vi "SetAttributeViString.vi"(7 "AttributeValue":string, 8 "error in (no error)":errorcluster {"code" format="%.0x"}, 9 "AttributeID":u32(ring)=1150015 items=["CALIBRATION_MESSAGE"=1150015, "CALIBRATION_SECURITY_CODE "=1150013, "DIGITIZER_MEMORY_MEASUREMENT_DATA_AUTO_SAVE_FILE"=1150071, "DISPLAY_TEXT"=1150017, "ROUTE_MONITOR_CHANNEL"=1150010, "SCAN_LIST"=1150004, "SYSTEM_DATE"=1150020, "SYSTEM_TIME"=1150021, "SYSTEM_TRACING_FILE_NAME"=1150042, "USB_MEMORY_DATA_FILE"=1150056, "USB_MEMORY_MEASUREMENTS_DATA_AUTO_SAVE_FILE"=1150058, "USB_MEMORY_SELECT_RECALL_AUTO_FILE"=1150053], 11 "instrument handle":refnum<k15>) -> (0 "error out":errorcluster {"code" format="%.0x"}, 3 "instrument handle out":refnum<k15>)   [LabVIEW 2020, in "Keysight DAQ970.lvlib"]
doc: "Sets a String attribute from the instrument driver.\nThe following Attributes are supported:\n\nCALIBRATION_MESSAGE\n\nCALIBRATION_SECURITY_CODE\n\nDIGITIZER_MEMORY_MEASUREMENT_DATA_AUTO_SAVE_FILE\n\nDISPLAY_TEXT\n\nROUTE_MONITOR_CHANNEL\n\nSCAN_LIST\n\nSYSTEM_DATE\n\nSYSTEM_TIME\n\nSYSTEM_TRACING_FILE_NAME\n\nUSB_MEMORY_DATA_FILE\n\nUSB_MEMORY_MEASUREMENTS_DATA_AUTO_SAVE_FILE\n\nUSB_MEMORY_SELECT_RECALL_AUTO_FILE"
uses:
  Keysight DAQ970.lvlib
  KtDAQ970.dll
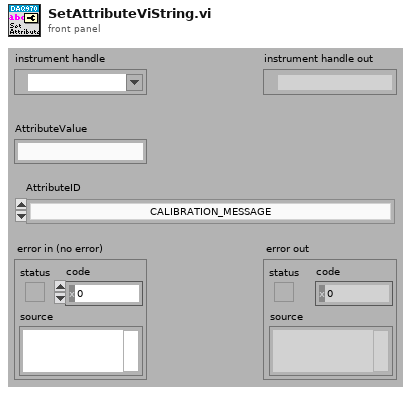
[diagram p1: front panel]
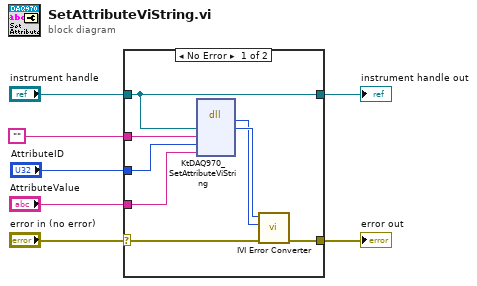
[diagram p0: block diagram]
diagram:
  n1 = case shown="No Error" "error in (no error)" {
    selector: "error in (no error)" -> [w13 w17]
    tunnel: [w12 w17] -> w7
    tunnel: "instrument handle" -> [w8 w16]
    tunnel: "" -> [w11 _]
    tunnel: "AttributeID" -> [w10 _]
    tunnel: "AttributeValue" -> [w9 _]
    tunnel: [w8 w16] -> w3
    frame No Error {
      n2 = dll-call lib="KtDAQ970**.dll" fn="KtDAQ970_SetAttributeViString"("Vi"=w8, "RepCapIdentifier"=w11, "AttributeID"=w10, "AttributeValue"=w9) -> ("return type"=w14:i32, "Vi"=w15:u32)  [unwired: 6 in, 2 out]
      n3 = call "IVI Error Converter.vi"("error in (no error)"=w13, "IVI error code (0)"=w14, "instrument handle"=w15) -> ("error out"=w12:errorcluster)  [unwired: 7 in, 1 out]
    }
    frame Error {
    }
  }
  "error out" <- w7
  "instrument handle out" <- w3
